vi "CloseFile.vi"(8 "error in (no error)":errorcluster, 11 "DataLogRaster in":refnum<class "DataLogRaster.lvclass">) -> (0 "error out":errorcluster, 3 "DataLogRaster out":refnum<class "DataLogRaster.lvclass">)   [LabVIEW 2018, in "DataLogRaster.lvclass"]
uses:
  DataLogRaster.lvclass
  DataLogRaster.lvclass/DataLogRaster.ctl
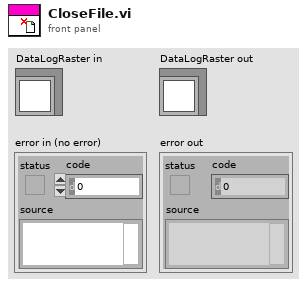
[diagram p1: front panel]
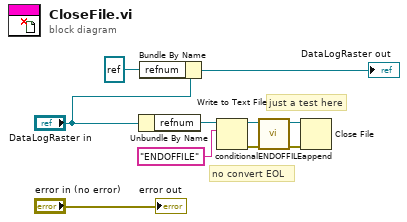
[diagram p0: block diagram]
diagram:
  # "just a test here"
  # "no convert EOL"
  n1 = Unbundle By Name("DataLogRaster in") -> ("refnum"=w4:refnum<file>)
  n2 = Bundle By Name(cluster="DataLogRaster in", "refnum"=refnum<file> refnum) -> (→"DataLogRaster out":refnum<class "DataLogRaster.lvclass">)
  n3 = Write to Text File(file (use dialog)=w4, text="ENDOFFILE") -> (refnum out=w6:refnum<file>, error out=w8:errorcluster)  [unwired: 2 in, 1 out]
  n4 = call "conditionalENDOFFILEappend.vi"("error in"=w8, "refnum"=w6) -> ("error out"=w9:errorcluster, "refnum out"=w7:refnum<file>)  [unwired: 8 in]
  n5 = Close File(refnum=w7, error in=w9) -> ()  [unwired: 2 out]
  "error out" <- "error in (no error)"
